vi "Is in HovaCAL fixed.vi"(11 "Komponente:":u16) -> (3 "is in HovaCAL fixed":bool)   [LabVIEW 2020, in "Linearisierung v2.lvlib" / "SpanEinstellungen.lvlib"]
uses:
  Gasteiler/Aktionen FGV Gasteiler Daten.ctl
  GasteilerType.ctl
  Gasteiler/HovaCAL_Interface/Kommunikation/Aktion FGV HovaCAL Interface Autolin.ctl
  SpanEinstellungen.lvlib
  Gasteiler/HovaCAL_Interface/Kommunikation/Kommunikation.lvlib
  Gasteiler/Gasteiler.lvlib
  Linearisierung v2.lvlib
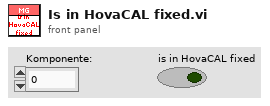
[diagram p1: front panel]
types:
  T1 = typedef "Linearisierung v2.lvlib/GasteilerType.ctl" = u16
  T2 = typedef "Linearisierung v2.lvlib/Gasteiler.lvlib/Aktionen FGV Gasteiler Daten.ctl" = enum16{"lesen", "Gasteiler Daten", "Seriellen Param.", "MB-Endwert", "laden", "speichern", "Anforderung", "TCP", "Aufzeichnung Start"}
  T3 = typedef "Linearisierung v2.lvlib/Gasteiler.lvlib/HovaCAL_Interface.lvlib/Kommunikation.lvlib/Aktion FGV HovaCAL Interface Autolin.ctl" = enum16{"lesen", "schreiben", "MFC Komponente fix setzen", "init"}
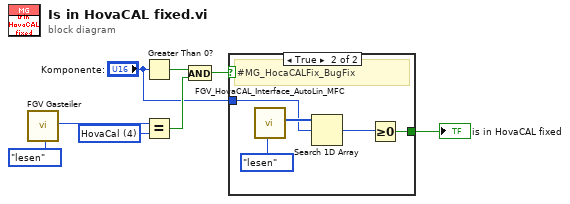
[diagram p0: block diagram]
diagram:
  w5 = T1 4 items=["LNI", "Analog-Display", "AVL GDU", "Horiba GDC", "HovaCal", "Horiba SGD 710C"] ("y")
  n1 = call "FGV Gasteiler.vi"("Aktionen"=Aktionen_FGV_Gasteiler_Daten."lesen") -> ("Gasteiler Type"=w6:T1)  [unwired: 11 in, 7 out]
  n2 = Greater Than 0?(x="Komponente:") -> (x > 0?=w8:bool)
  n3 = Equal?(x=w6, y=w5) -> (x = y?=w3:bool)
  n4 = And(x=w8, y=w3) -> (x .and. y?=w4:bool)
  n5 = case shown="True" w4 {
    tunnel: "Komponente:" -> [_ w11]
    tunnel: [_ w9] -> w1
    frame False {
    }
    frame True {
      # "#MG_HocaCALFix_BugFix"
      n6 = call "FGV_HovaCAL_Interface_AutoLin_MFC.vi"("Aktion"=Aktion_FGV_HovaCAL_Interface_Autolin."lesen") -> ("MFV Komponente fix out"=w12:u16[])  [unwired: 7 in, 3 out]
      n7 = Search 1D Array(1D array=w12, element=w11) -> (index of element=w10:i32)  [unwired: 1 in]
      n8 = Greater Or Equal To 0?(x=w10) -> (x >= 0?=w9:bool)
    }
  }
  "is in HovaCAL fixed" <- w1
